vi "Create Sysdef Tree from Parameters Clusters.vi"(8 "error in":errorcluster, 10 "Channels":T1[](array[typedef]), 11 "Device Ptr":u64) -> (0 "error out":errorcluster, 3 "Device Ptr dup":u64)   [LabVIEW 2017, in "Ballard Arinc-429 System Explorer.lvlib"]
uses:
  Ballard Arinc-429 System Explorer.lvlib
  Parse Parameters File/XML_Channel.ctl
  Parse Parameters File/XML_Label.ctl
  Parse Parameters File/XML_Parameter.ctl
  <vilib>/NI Veristand/Custom Device Tools/Custom Device Utility Library/NI VeriStand - Search for Item by GUID.vi
  Shared/Controls and Global/Global.vi
  <vilib>/NI Veristand/Custom Device API/NI VeriStand - Get Item Property.vi
  <vilib>/NI Veristand/Custom Device API/Get Item Property (U32).vi
  <vilib>/NI Veristand/Custom Device API/NI VeriStand - Get Item Children.vi
  <vilib>/NI Veristand/Custom Device API/Get Item Property (U16).vi
  <vilib>/NI Veristand/Custom Device Tools/Custom Device Utility Library/NI VeriStand - Search for All Items by GUID.vi
  Shared/Ballard Arinc-429 Shared.lvlib
  <vilib>/NI Veristand/Custom Device Tools/Custom Device Utility Library/Custom Device Utility Library.lvlib
  <vilib>/NI Veristand/Custom Device API/Custom Device API.lvlib
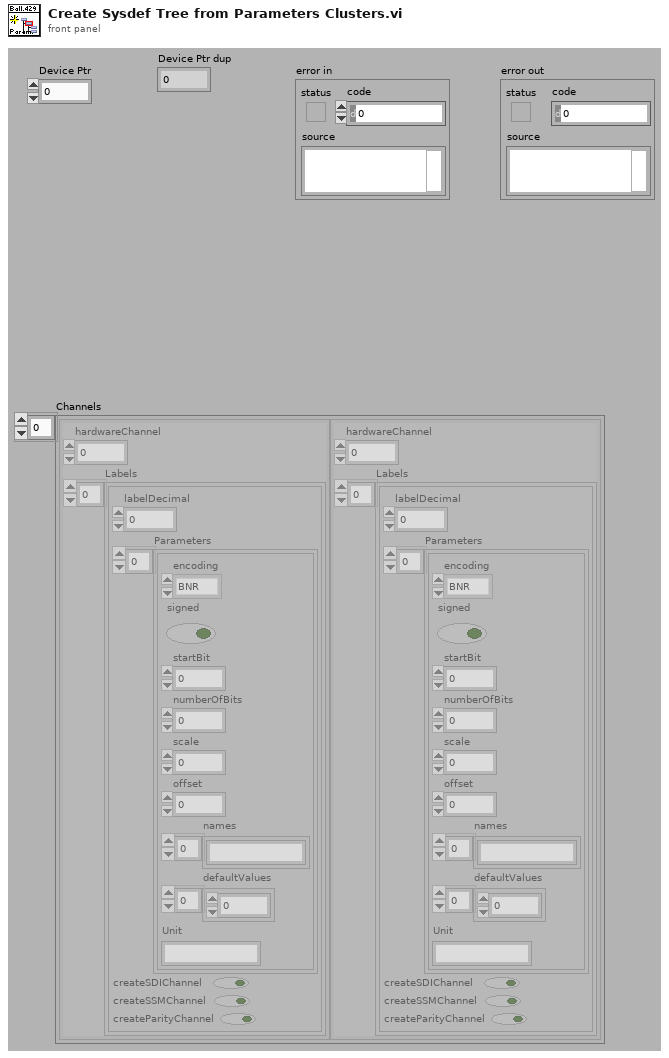
[diagram p1: front panel]
types:
  T1 = typedef "XML_Channel.ctl" = cluster{"hardwareChannel":i32, "Labels":T2[]}
  T2 = typedef "XML_Label.ctl" = cluster{"labelDecimal":i32, "Parameters":T3[], "createSDIChannel":bool, "createSSMChannel":bool, "createParityChannel":bool}
  T3 = typedef "XML_Parameter.ctl" = cluster{"encoding":enum16{"BNR", "BCD", "Discrete"}, "signed":bool, "startBit":i32, "numberOfBits":i32, "scale":dbl, "offset":dbl, "names":string[], "defaultValues":dbl[], "Unit":string}
  T4 = typedef "Custom Device API.lvlib/Custom Device Item Ref.ctl" = u64
  T5 = typedef "Custom Device API.lvlib/Custom Device Item Info.ctl" = cluster{"Name":string, "Is Channel":bool, "GUID":string, "Is Waveform":bool}
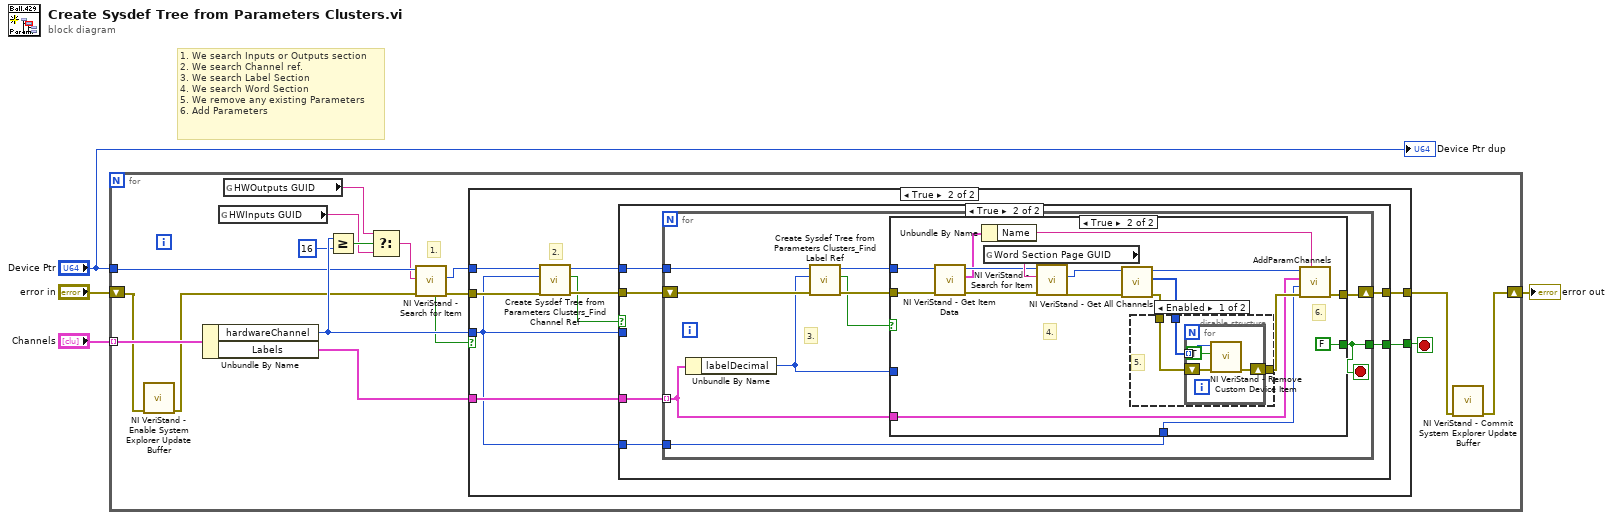
[diagram p0: block diagram]
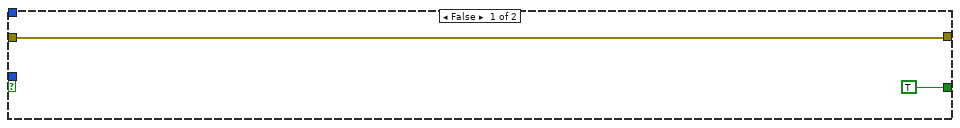
[diagram p2: hidden frame]
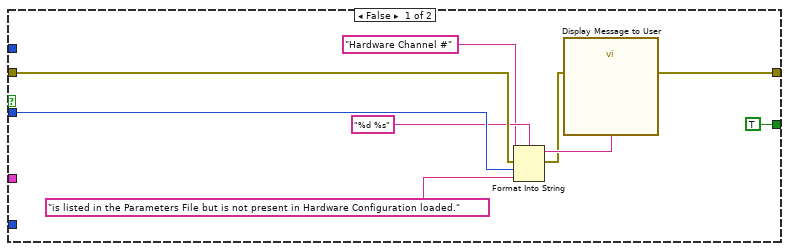
[diagram p3: hidden frame]
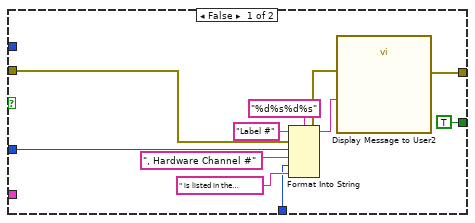
[diagram p4: hidden frame]
diagram:
  # "1. We search Inputs or Outputs section\n2. We search Channel ref.\n3. We search Label Section\n4. We search Word Section\n5. We remove any existing Parameters\n6. Add Parameters"
  n1 = for {
    tunnel: "Device Ptr" -> [w16]
    shift-right: [w5] -> w2
    shift-left: "error in" -> [w8]
    tunnel: "Channels" -> [w21] mode=indexing
    stop <- w9 stop-if-true
    # "1."
    n2 = call <vilib>:"NI VeriStand - Enable System Explorer Update Buffer.vi"("error in (no error)"=w8) -> ("error out"=w7:errorcluster)  [unwired: 10 in]
    n3 = Unbundle By Name(w21) -> ("hardwareChannel"=w19:i32, "Labels"=w20:T2[])
    n4 = global read "Global.vi" "HWInputs GUID"() -> (w11:string)
    n5 = global read "Global.vi" "HWOutputs GUID"() -> (w12:string)
    n6 = Greater Or Equal?(x=w19, y=16) -> (x >= y?=w17:bool)
    n7 = Select(t=w12, s=w17, f=w11) -> (s? t:f=w10:string)
    n8 = call-poly <vilib>:"NI VeriStand - Search for Item.vi"("error in"=w7, "Item GUID"=w10, "Section Ref in"=w16) -> ("error out"=w13:errorcluster, "Item Ref"=w15:T4, "Found"=w14:bool)  [unwired: 5 in, 1 out]
    n9 = case shown="True" w14 {
      tunnel: [w23 w32] -> w6
      tunnel: w20 -> [_ w29]
      tunnel: w19 -> [_ w25]
      tunnel: w15 -> [_ w24]
      tunnel: w13 -> [w23 w27]
      tunnel: [TRUE w26] -> w9
      frame False {
      }
      frame True {
        # "2."
        n10 = call "Create Sysdef Tree from Parameters Clusters_Find Channel Ref.vi"("error in (no error)"=w27, "hardwareChannel"=w25, "Item Ref in"=w24) -> ("error out"=w31:errorcluster, "Found"=w30:bool, "Item Ref out"=w28:T4)  [unwired: 6 in]
        n11 = case shown="True" w30 {
          tunnel: [w41 w45] -> w32
          tunnel: w31 -> [w40 w47]
          tunnel: w28 -> [_ w42]
          tunnel: w25 -> [w37 _]
          tunnel: w29 -> [_ w46]
          tunnel: w25 -> [_ w44]
          tunnel: [TRUE w43] -> w26
          frame False {
            n12 = Format Into String(format string="%d %s", initial string="Hardware Channel #", error in=w40, w37, "is listed in the Parameters File but is not present in Hardware Configuration loaded." ("initial string")) -> (resulting string=w39:string, error out=w38:errorcluster)
            n13 = call "Display Message to User"("error in (no error)"=w38, "Message"=w39) -> ("error out"=w41:errorcluster)  [unwired: 8 in, 1 out]
          }
          frame True {
            n14 = for {
              tunnel: w42 -> [w53]
              tunnel: w46 -> [w56] mode=indexing
              shift-right: [w57] -> w45
              shift-left: w47 -> [w52]
              tunnel: w44 -> [w55]
              tunnel: [w54] -> w43
              stop <- w54 stop-if-true
              # "3."
              n15 = Unbundle By Name(w56) -> ("labelDecimal"=w50:i32)
              n16 = call "Create Sysdef Tree from Parameters Clusters_Find Label Ref.vi"("error in (no error)"=w52, "decimalLabel"=w50, "Item Ref in"=w53) -> ("error out"=w51:errorcluster, "Found"=w48:bool, "Item Ref out"=w49:T4)  [unwired: 6 in]
              n17 = case shown="True" w48 {
                tunnel: w51 -> [w61 w76]
                tunnel: w49 -> [_ w69]
                tunnel: [w63 w78] -> w57
                tunnel: w56 -> [_ w77]
                tunnel: w50 -> [w66 _]
                tunnel: w55 -> [w59 w71]
                tunnel: [TRUE FALSE] -> w54
                frame False {
                  n18 = Format Into String(format string="%d%s%d%s", initial string="Label #", error in=w61, w66, ", Hardware Channel #" ("initial string"), w59, " is listed in the Parameters File but is not present in Hardware Configuration loaded." ("initial string")) -> (resulting string=w62:string, error out=w60:errorcluster)
                  n19 = call "Display Message to User2"("error in (no error)"=w60, "Message"=w62) -> ("error out"=w63:errorcluster)  [unwired: 8 in, 1 out]
                }
                frame True {
                  # "6."
                  # "4."
                  n20 = call <vilib>:"NI VeriStand - Get Item Data.vi"("error in (no error)"=w76, "Item Ref in"=w69) -> ("error out"=w74:errorcluster, "Item Info"=w73:T5, "Item Ref out"=w75:T4)  [unwired: 6 in, 1 out]
                  n21 = Unbundle By Name(w73) -> ("Name"=w72:string)
                  n22 = global read "Global.vi" "Word Section Page GUID"() -> (w85:string)
                  n23 = call-poly <vilib>:"NI VeriStand - Search for Item.vi"("error in"=w74, "Item GUID"=w85, "Section Ref in"=w75) -> ("error out"=w83:errorcluster, "Item Ref"=w84:T4)  [unwired: 5 in, 2 out]
                  n24 = call <vilib>:"NI VeriStand - Get All Channels.vi"("error in"=w83, "Section Ref in"=w84) -> ("error out"=w81:errorcluster, "Channel Refs"=w82:T4[], "Section Ref out"=w80:T4)  [unwired: 6 in, 1 out]
                  n25 = disable-structure shown="Enabled" {
                    disable-tunnel: w82 -> [w88 _]
                    disable-tunnel: w81 -> [w87 w93]
                    disable-tunnel: [w86 w93] -> w79
                    frame Enabled {
                      # "5."
                      n26 = for {
                        tunnel: w88 -> [w92] mode=indexing
                        shift-right: [w90] -> w86
                        shift-left: w87 -> [w91]
                        n27 = call <vilib>:"NI VeriStand - Remove Custom Device Item.vi"("error in (no error)"=w91, "Force Delete (F)"=TRUE, "Item Ref in"=w92) -> ("error out"=w90:errorcluster)  [unwired: 7 in, 1 out]
                      }
                    }
                    frame Disabled {
                    }
                  }
                  n28 = call "AddParamChannels.vi"("Label Name"=w72, "error in"=w79, "HardwareChannel"=w71, "Label Parameters"=w77, "Node Ref In"=w80) -> ("error out"=w78:errorcluster)  [unwired: 5 in, 1 out]
                }
              }
            }
          }
        }
      }
    }
    n29 = call <vilib>:"NI VeriStand - Commit System Explorer Update Buffer.vi"("error in (no error)"=w6) -> ("error out"=w5:errorcluster)  [unwired: 10 in]
  }
  "error out" <- w2
  "Device Ptr dup" <- "Device Ptr"
